vi "Encoder Operation.vi"(6 "Loop Time(ms)":u32=10, 7 "Enc":tag="A/ENC", 8 "error in (no error)":errorcluster, 9 "Init-Enc-Pos":dbl, 10 "Reset Counter":bool, 11 "Enc-Coefficient":dbl=0.1) -> (0 "error out":errorcluster, 1 "Velocity(rad/s)":dbl, 2 "Velocity(deg/s)":dbl, 3 "Pos Passed(deg)":dbl, 4 "Counter Value":dbl)   [LabVIEW 2013, in "SGDV_Ctrl_v13_lib.lvlib"]
uses:
  SGDV_Ctrl_v13_lib.lvlib
  <vilib>/myRIO/Common/Instrument Driver Framework/myRIO v1.0/Encoder/typedefs/Encoder Signal Mode.ctl
  <vilib>/myRIO/Instrument Drivers/Onboard IO/Encoder/vis/Open.vi
  <vilib>/myRIO/Common/Instrument Driver Framework/myRIO v1.0/Encoder/vis/myRIO v1.1 Open Encoder.vi
  <vilib>/myRIO/Common/Instrument Driver Framework/myRIO v1.0/Encoder/vis/myRIO v1.0 Close Encoder.vi
  <vilib>/myRIO/Common/Instrument Driver Framework/myRIO v1.0/Encoder/vis/myRIO v1.2 Open Encoder.vi
  <vilib>/myRIO/Common/Instrument Driver Framework/Utilities/vis/Validate Channels.vi
  <vilib>/myRIO/Common/Instrument Driver Framework/myRIO v1.0/Encoder/vis/myRIO v1.0 Reserve Encoder.vi
  <vilib>/myRIO/Common/Instrument Driver Framework/myRIO v1.0/Encoder/vis/myRIO v1.0 Unreserve Encoder.vi
  <vilib>/myRIO/Common/Instrument Driver Framework/myRIO v1.0/Encoder/vis/myRIO v1.0 Build MUX Configuration Encoder.vi
  <vilib>/myRIO/Common/Instrument Driver Framework/myRIO v1.0/Resource Manager/vis/myRIO v1.0 Reserve Channel List.vi
  <vilib>/myRIO/Common/Instrument Driver Framework/myRIO v1.0/Resource Manager/vis/myRIO v1.0 Unreserve Channel List.vi
  <vilib>/myRIO/Common/Instrument Driver Framework/myRIO v1.0/Resource Manager/vis/myRIO v1.0 Create Configuration List.vi
  <vilib>/myRIO/Common/Instrument Driver Framework/myRIO v1.0/Resource Manager/vis/myRIO v1.0 Reserve Channel.vi
  <vilib>/myRIO/Common/Instrument Driver Framework/myRIO v1.0/Resource Manager/vis/myRIO v1.0 Unreserve Channel.vi
  <vilib>/myRIO/Common/Instrument Driver Framework/myRIO v1.0/Resource Manager/vis/myRIO v1.0 Build Mutex Name.vi
  <vilib>/myRIO/Common/Instrument Driver Framework/Utilities/vis/Set_Get Target Info.vi
  <vilib>/Utility/error.llb/Error Cluster From Error Code.vi
  <vilib>/myRIO/Common/Instrument Driver Framework/myRIO v1.0/Encoder/vis/myRIO v1.0 Configure Encoder.vi
  <vilib>/myRIO/Common/Instrument Driver Framework/myRIO v1.0/myRIO v1.1 Open.vi
  <vilib>/Utility/VariantDataType/GetNumericInfo.vi
  <vilib>/myRIO/Common/Instrument Driver Framework/Utilities/vis/IO Manager.vi
  <vilib>/myRIO/Common/Instrument Driver Framework/Utilities/vis/Configuration Manager.vi
  <vilib>/myRIO/Common/Instrument Driver Framework/myRIO v1.0/Resource Manager/vis/myRIO v1.0 Configure IO.vi
  <vilib>/myRIO/Common/Instrument Driver Framework/myRIO v1.0/myRIO v1.0 Close.vi
  <vilib>/myRIO/Common/Instrument Driver Framework/myRIO v1.0/Encoder/vis/myRIO v1.0 Shutdown Encoder.vi
  <vilib>/myRIO/Common/Instrument Driver Framework/myRIO v1.0/myRIO v1.2 Open.vi
  <vilib>/myRIO/Common/Instrument Driver Framework/myRIO v1.0/Encoder/vis/myRIO v1.0 Read Encoder.vi
  <vilib>/ptbypt/NI_PtbyPt.lvlib
  <vilib>/myRIO/Instrument Drivers/Onboard IO/Encoder/Encoder.lvlib
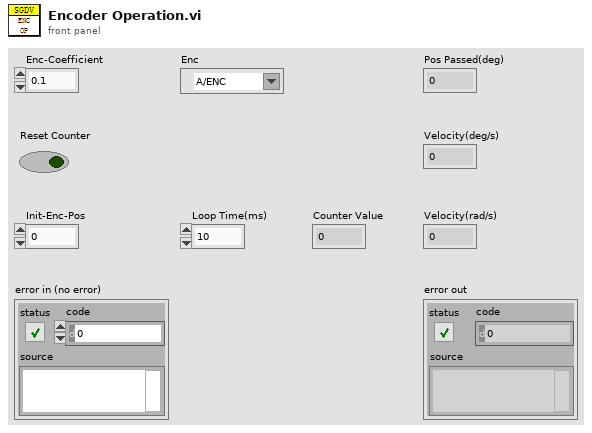
[diagram p1: front panel]
types:
  T1 = typedef "Encoder Signal Mode.ctl" = enum16{"Quadrature Phase Signal", "Step and Direction Signal"}
  T2 = typedef "Encoder.lvlib/Encoder Reference.ctl" = cluster{"myRIO Reference":T3, "Encoder Channels Enum":T7}
  T3 = typedef "myRIO Generic Hardware Reference.ctl" = cluster{"myRIO Model":T4, "myRIO Hardware Reference":T5}
  T4 = typedef "Hardware Version Enum.ctl" = enum16{"Unknown", "myRIO-1900", "myRIO-1950"}
  T5 = typedef "myRIO v1.0 Reference.ctl" = cluster{"Generic FPGA Reference":T6, "Allow multiple opens":bool}
  T6 = typedef "Generic FPGA Reference.ctl" = refnum<k20>
  T7 = typedef "Encoder Channels Enum.ctl" = enum16{"Not Connected", "C/ENC0", "C/ENC1", "A/ENC", "B/ENC"}
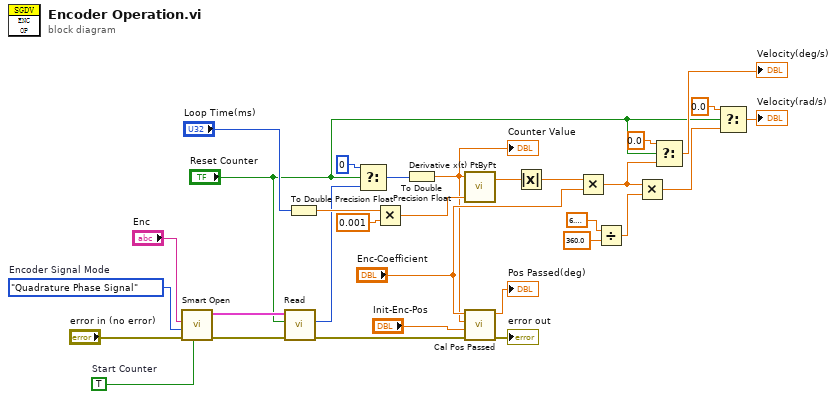
[diagram p0: block diagram]
diagram:
  w8 = TRUE  # Start Counter
  w9 = Encoder_Signal_Mode."Quadrature Phase Signal"  # Encoder Signal Mode
  n1 = call <vilib>:"Smart Open.vi"("Start Counter"=w8, "error in (no error)"="error in (no error)", "Encoder Signal Mode"=w9, "Channel Name"="Enc") -> ("error out"=w6:errorcluster, "Encoder Ref Out"=w7:T2)  [unwired: 6 in]
  n2 = call <vilib>:"Read.vi"("error in (no error)"=w6, "Reset Counter"="Reset Counter", "Encoder Ref In"=w7) -> ("error out"=w4:errorcluster, "Counter Value"=w2:i32)  [unwired: 4 in, 3 out]
  n3 = To Double Precision Float(number="Loop Time(ms)") -> (double precision float=w31:dbl)
  n4 = Select(t=0, s="Reset Counter", f=w2) -> (s? t:f=w15:i32)
  n5 = Multiply(x=w31, y=0.001) -> (x*y=w29:dbl)
  n6 = To Double Precision Float(number=w15) -> (double precision float=w11:dbl)
  "Counter Value" <- w11
  n7 = call <vilib>:"Derivative x(t) PtByPt.vi"("dt"=w29, "x"=w11) -> ("dx/dt"=w24:dbl)  [unwired: 2 in, 1 out]
  n8 = call "Cal Pos Passed.vi"("error in (no error)"=w4, "Init-Enc-Pos(cnt)"="Init-Enc-Pos", "Current-Enc-Pos(cnt)"=w11, "Enc-Coefficient"="Enc-Coefficient") -> ("error out"=→"error out":errorcluster, "Pos Passed(deg)"=→"Pos Passed(deg)":dbl)  [unwired: 6 in]
  n9 = Absolute Value(x=w24) -> (abs(x)=w23:dbl)
  n10 = Multiply(x=w23, y="Enc-Coefficient") -> (x*y=w21:dbl)
  n11 = Divide(x=6.283185307179586, y=360.0) -> (x/y=w25:dbl)
  n12 = Multiply(x=w21, y=w25) -> (x*y=w19:dbl)
  n13 = Select(t=0.0, s="Reset Counter", f=w21) -> (s? t:f=→"Velocity(deg/s)":dbl)
  n14 = Select(t=0.0, s="Reset Counter", f=w19) -> (s? t:f=→"Velocity(rad/s)":dbl)
